vi "Agilent_read.vi"(0 "VISA resource name":refnum<visa-resource-name>, 1 "error in (no error)":errorcluster) -> (2 "VISA resource name out":refnum<visa-resource-name>, 3 "Output current":dbl, 4 "Output Voltage":dbl, 5 "error out":errorcluster)   [LabVIEW 2017]
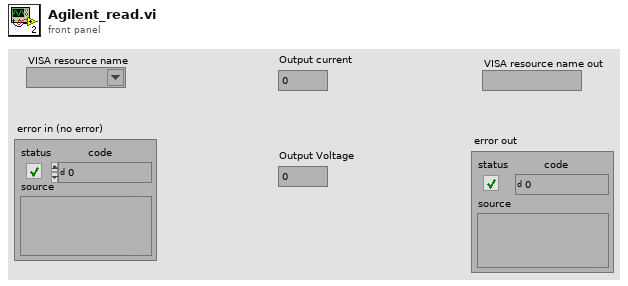
[diagram p1: front panel]
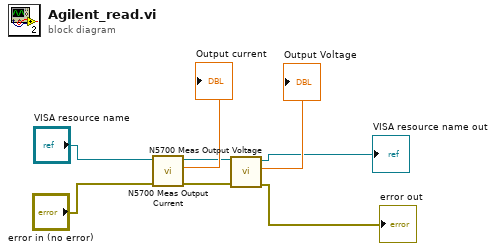
[diagram p0: block diagram]
diagram:
  n1 = call <instrlib>:"N5700 Meas Output Current.vi"("error"="error in (no error)", "VISA"="VISA resource name") -> ("error out"=w3:errorcluster, "Output Current"=→"Output current":dbl, "VISA out"=w6:refnum<visa-resource-name>)  [unwired: 4 in]
  n2 = call <instrlib>:"N5700 Meas Output Voltage.vi"("error"=w3, "VISA"=w6) -> ("error out"=→"error out":errorcluster, "Output Voltage"=→"Output Voltage":dbl, "VISA out"=→"VISA resource name out":refnum<visa-resource-name>)  [unwired: 4 in]
